vi "Logging Message Loop.vi"(8 "error in (no error)":errorcluster, 10 "Data Queue":refnum<queue>, 11 "Message Queues":T1) -> (0 "error out":errorcluster)   [LabVIEW 2023, in "Logging.lvlib"]
doc: "The message loop subVI to handle messages pertaining to logging data."
uses:
  Logging.lvlib
  support/Message Queue/All Message Queues.ctl
  support/Message Queue/Message Cluster.ctl
  Logging Configuration.ctl
  Logging State.ctl
  support/Message Queue/Enqueue Message (Single).vi
  <vilib>/Utility/error.llb/Error Cluster From Error Code.vi
  <vilib>/ErrorRing/Error Ring.xnode
  <vilib>/addons/_JKI.lib/REST Client/classes/REST Client/REST Client.lvclass
  support/Message Queue/Message Queue.lvlib
  <vilib>/addons/_JKI.lib/Serialization/JSON/JKI JSON Serialization.lvlib
panel:
  in  "CardId":string
  in  "City":string
  in  "Country":string="Poland"
  in  "FastAPI write route":string="/write_api"
  in  "FastAPI URI":string="http://localhost:80"
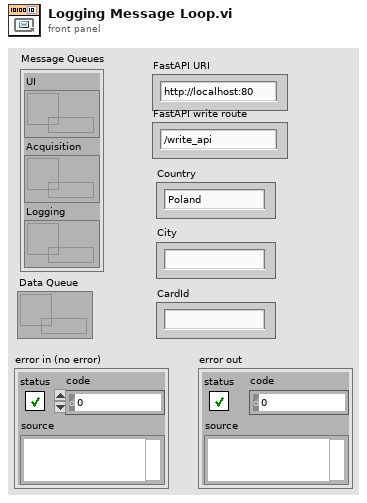
[diagram p1: front panel]
types:
  T1 = typedef "Message Queue.lvlib/All Message Queues.ctl" = cluster{"UI":refnum<queue>, "Acquisition":refnum<queue>, "Logging":refnum<queue>}
  T2 = typedef "Logging.lvlib/Logging Configuration.ctl" = cluster{"Log File Base Path":path, "TDMS File Reference":refnum<k34>}
  T3 = typedef "Logging.lvlib/Logging State.ctl" = enum16{"Idle", "Logging"}
  T4 = enum16{"open", "open or create", "create or replace", "create", "open (read-only)"}
  T5 = cluster{"Array":waveform(dbl)[], "Country":string, "City":string, "CardId":string}
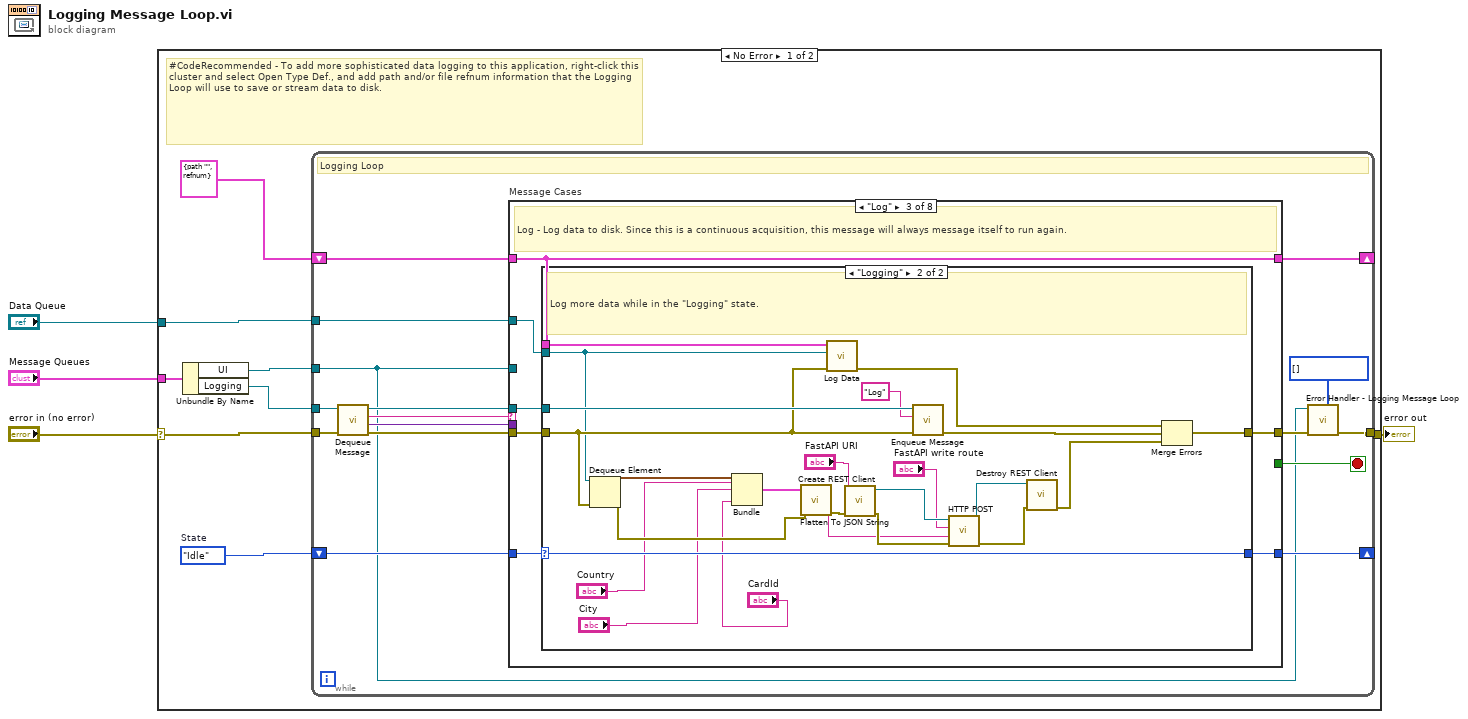
[diagram p0: block diagram]
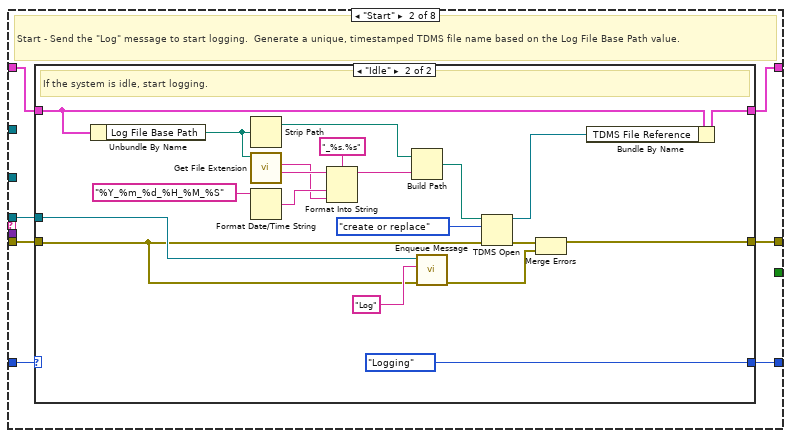
[diagram p3: hidden frame]
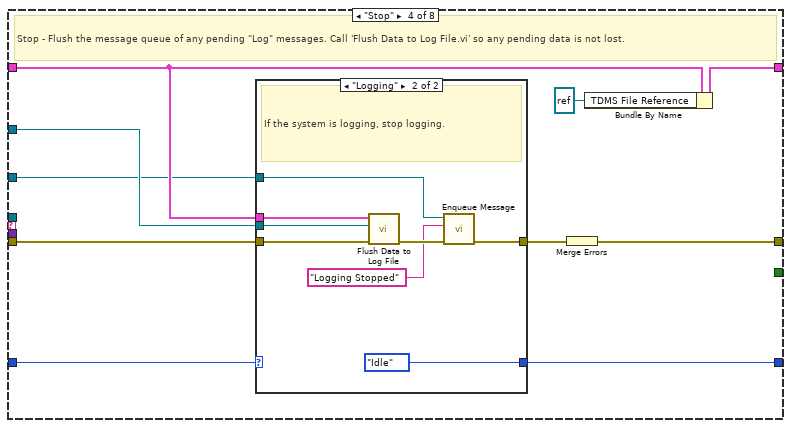
[diagram p6: hidden frame]
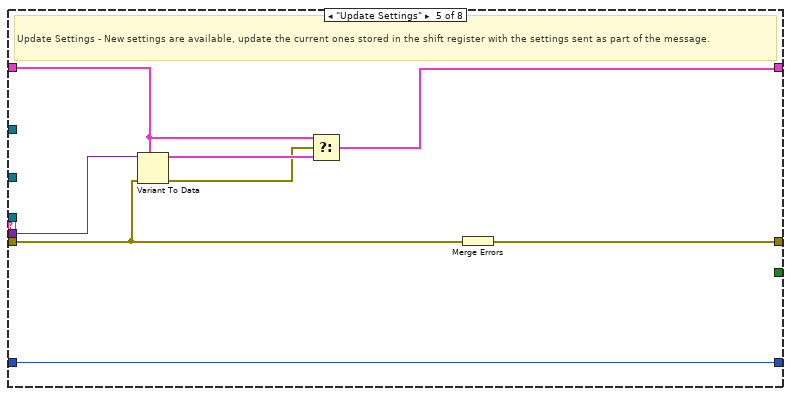
[diagram p8: hidden frame]
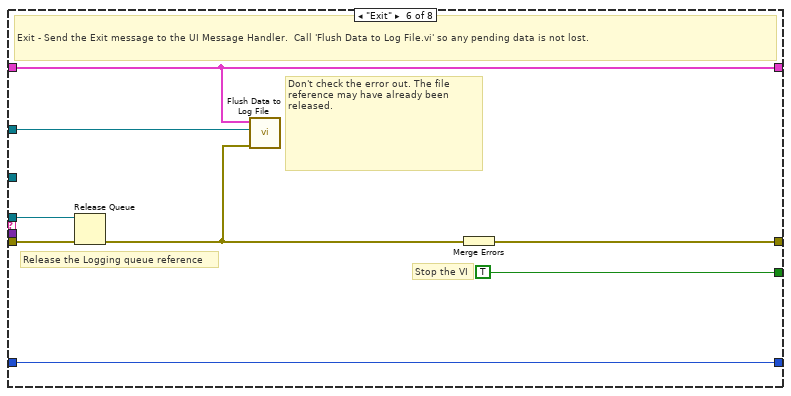
[diagram p9: hidden frame]
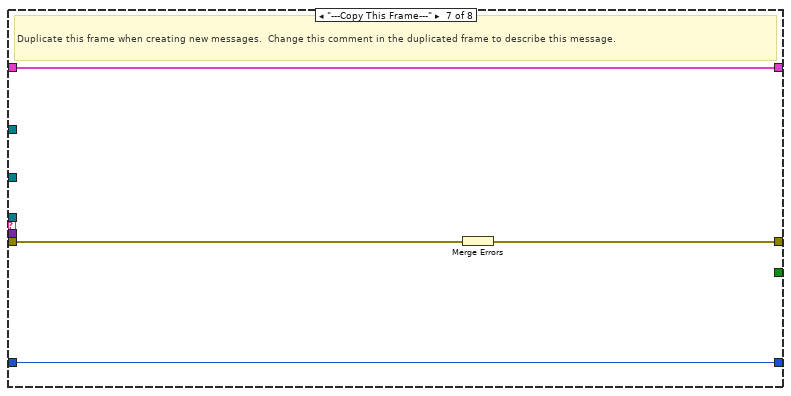
[diagram p10: hidden frame]
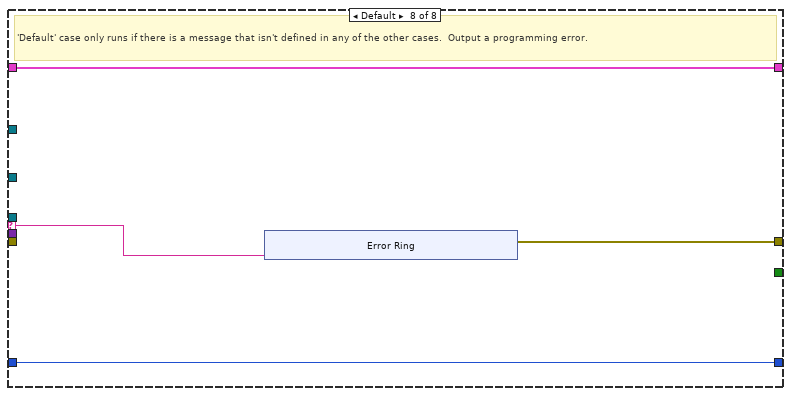
[diagram p11: hidden frame]
diagram:
  n1 = case shown="No Error" "error in (no error)" {
    selector: "error in (no error)" -> [w8 w146]
    tunnel: "Message Queues" -> [w12 _]
    tunnel: [w10 w146] -> w3
    tunnel: "Data Queue" -> [w7 _]
    frame No Error {
      w5 = Logging_State."Idle"  # State
      # "#CodeRecommended - To add more sophisticated data logging to this application, right-click this cluster and select Open Type Def., and add path and/or file refnum information that the Logging Loop will use to save or stream data to disk."
      n2 = Unbundle By Name(w12) -> ("UI"=w6:refnum<queue>, "Logging"=w11:refnum<queue>)
      n3 = while {
        tunnel: w11 -> [w20]
        shift-right: [w27] -> _
        shift-left: T2 {"Log File Base Path"=path "", "TDMS File Reference"=refnum} ("Logging Configuration") -> [w28]
        tunnel: w6 -> [w14]
        tunnel: w7 -> [w19]
        shift-right: [w17] -> _
        shift-left: w5 -> [w18]
        tunnel: w8 -> [w25]
        tunnel: [w16] -> w10
        stop <- w26 stop-if-true
        # "Logging Loop"
        n4 = call "Dequeue Message.vi"("error in (no error)"=w25, "Message Queue"=w20) -> ("error out"=w24:errorcluster, "Message Data"=w22:variant, "Message"=w23:string, "dup Message Queue"=w21:refnum<queue>)  [unwired: 6 in]
        n5 = case "Message Cases" shown="\"Log\"" w23 {
          selector: w23 -> [_ _ _ _ _ _ _ w135]
          tunnel: w21 -> [_ w37 w67 _ _ w127 _ _]
          tunnel: w24 -> [w30 w36 w65 w98 w116 w128 w134 _]
          tunnel: [w30 w38 w68 w104 w122 w129 w132 w136] -> w15
          tunnel: w28 -> [w31 w35 w64 w99 w120 w125 w133 w138]
          tunnel: [w31 w34 w64 w102 w117 w125 w133 w138] -> w27
          tunnel: [_ _ _ _ _ TRUE _ _] -> w26
          tunnel: w22 -> [_ _ _ _ w121 _ _ _]
          tunnel: w14 -> [_ _ _ w95 _ _ _ _]
          tunnel: w19 -> [_ _ w66 w100 _ w124 _ _]
          tunnel: w18 -> [w29 w33 w63 w97 w115 w123 w131 w137]
          tunnel: [w29 w32 w62 w96 w115 w123 w131 w137] -> w17
          frame "Initialize" {
            # "Initialize - gets called when first launched. Currently a no-op."
          }
          frame "Start" {
            # "Start - Send the \"Log\" message to start logging.  Generate a unique, timestamped TDMS file name based on the Log File Base Path value."
            n6 = case shown="\"Idle\"" w33 {
              selector: w33 -> [w40 _]
              tunnel: [w39 w43] -> w38
              tunnel: w37 -> [_ w44]
              tunnel: w36 -> [w39 w42]
              tunnel: w35 -> [w41 w45]
              tunnel: [w41 w47] -> w34
              tunnel: [w40 Logging_State."Logging" ("State")] -> w32
              frame "Logging" {
                # "The system is already logging. Ignore the \"Start\" message."
              }
              frame "Idle" {
                # "If the system is idle, start logging."
                n7 = Unbundle By Name(w45) -> ("Log File Base Path"=w60:path)
                n8 = Strip Path(path=w60) -> (stripped path=w57:path)  [unwired: 1 out]
                n9 = call <vilib>:"Get File Extension.vi"("file"=w60) -> ("filename without extension"=w58:string, "lowercase file extension"=w54:string)  [unwired: 6 in, 3 out]
                n10 = Format Date/Time String(time format string (%c)="%Y_%m_%d_%H_%M_%S") -> (date/time string=w55:string)  [unwired: 2 in]
                n11 = Format Into String(format string="_%s.%s", initial string=w58, w55, w54) -> (resulting string=w53:string)  [unwired: 1 in, 1 out]
                n12 = Build Path(base path=w57, name or relative path=w53) -> (appended path=w52:path)
                n13 = call-poly "Enqueue Message.vi"("error in (no error)"=w42, "Message"="Log", "Message Queue"=w44) -> ("error out"=w50:errorcluster)  [unwired: 7 in, 1 out]
                n14 = TDMS Open(8:w42, 10:T4."create or replace" ("operation (0:open)"), 11:w52) -> (0:w51:errorcluster, 3:w48:refnum<k34>)  [unwired: 4 in]
                n15 = Merge Errors(w51, w50) -> (w43:errorcluster)
                n16 = Bundle By Name(cluster=w45, "TDMS File Reference"=w48) -> (w47:T2)
              }
            }
          }
          frame "Log" {
            # "Log - Log data to disk. Since this is a continuous acquisition, this message will always message itself to run again."
            n17 = case shown="\"Logging\"" w63 {
              selector: w63 -> [w70 w88]
              tunnel: [w69 w94] -> w68
              tunnel: w67 -> [_ w92]
              tunnel: w66 -> [_ w83]
              tunnel: w65 -> [w69 w84]
              tunnel: w64 -> [_ w89]
              tunnel: [w70 w88] -> w62
              frame "Idle" {
                # "Ignore \"Log\" messages when the logging is idle."
              }
              frame "Logging" {
                # "Log more data while in the \"Logging\" state."
                n18 = Dequeue Element(queue=w83, error in (no error)=w84) -> (element=w75:waveform(dbl)[], error out=w76:errorcluster)  [unwired: 1 in, 2 out]
                n19 = Bundle("Array"=w75, "Country"="Country", "City"="City", "CardId"="CardId") -> (w74:T5)  [unwired: 1 in]
                n20 = call <vilib>:"Flatten To JSON String.vi"("error in (no error)"=w76, "Variant"=w74) -> ("error out"=w82:errorcluster, "JSON String"=w81:string)  [unwired: 8 in]
                n21 = call "Log Data.vi"("error in (no error)"=w84, "Data Queue"=w83, "Logging Configuration"=w89) -> ("error out"=w91:errorcluster)  [unwired: 8 in]
                n22 = call <vilib>:"Create REST Client.vi"("error in (no error)"=w82, "Base URL"="FastAPI URI") -> ("error out"=w85:errorcluster, "REST Client out"=w79:refnum<class "REST Client.lvclass">)  [unwired: 8 in]
                n23 = call-poly "Enqueue Message.vi"("error in (no error)"=w84, "Message"="Log", "Message Queue"=w92) -> ("error out"=w93:errorcluster)  [unwired: 7 in, 1 out]
                n24 = call-dynamic "HTTP POST.vi"("error in (no error)"=w85, "Request body"=w81, "Path"="FastAPI write route", "REST Client in"=w79) -> ("error out"=w86:errorcluster, "REST Client out"=w80:refnum<class "REST Client.lvclass">)  [unwired: 2 in, 4 out]
                n25 = call-dynamic "Destroy REST Client.vi"("error in (no error)"=w86, "REST Client in"=w80) -> ("error out"=w87:errorcluster)  [unwired: 9 in]
                n26 = Merge Errors(w91, w93, w87) -> (w94:errorcluster)
              }
            }
          }
          frame "Stop" {
            # "Stop - Flush the message queue of any pending \"Log\" messages. Call 'Flush Data to Log File.vi' so any pending data is not lost."
            n27 = case shown="\"Logging\"" w97 {
              selector: w97 -> [w105 _]
              tunnel: [w106 w109] -> w103
              tunnel: w100 -> [_ w113]
              tunnel: w99 -> [_ w112]
              tunnel: w98 -> [w106 w111]
              tunnel: [w105 Logging_State."Idle" ("State")] -> w96
              tunnel: w95 -> [_ w108]
              frame "Idle" {
                # "The system is already idle. Ignore the \"Stop\" message."
              }
              frame "Logging" {
                # "If the system is logging, stop logging."
                n28 = call "Flush Data to Log File.vi"("error in (no error)"=w111, "Data Queue"=w113, "Logging Configuration"=w112) -> ("error out"=w114:errorcluster)  [unwired: 8 in]
                n29 = call-poly "Enqueue Message.vi"("error in (no error)"=w114, "Message"="Logging Stopped", "Message Queue"=w108) -> ("error out"=w109:errorcluster)  [unwired: 7 in, 1 out]
              }
            }
            n30 = Merge Errors(w103) -> (w104:errorcluster)
            n31 = Bundle By Name(cluster=w99, "TDMS File Reference"=refnum<k34> refnum) -> (w102:T2)
          }
          frame "Update Settings" {
            # "Update Settings - New settings are available, update the current ones stored in the shift register with the settings sent as part of the message."
            n32 = Variant To Data(error in=w116, type=w120, Variant=w121) -> (data=w119:T2, error out=w118:errorcluster)
            n33 = Select(t=w120, s=w118, f=w119) -> (s? t:f=w117:T2)
            n34 = Merge Errors(w116) -> (w122:errorcluster)
          }
          frame "Exit" {
            # "Don't check the error out. The file reference may have already been released."
            # "Release the Logging queue reference"
            # "Stop the VI"
            # "Exit - Send the Exit message to the UI Message Handler.  Call 'Flush Data to Log File.vi' so any pending data is not lost."
            n35 = Release Queue(queue=w127, error in (no error)=w128) -> (error out=w126:errorcluster)  [unwired: 1 in, 2 out]
            n36 = call "Flush Data to Log File.vi"("error in (no error)"=w126, "Data Queue"=w124, "Logging Configuration"=w125) -> ()  [unwired: 8 in, 1 out]
            n37 = Merge Errors(w126) -> (w129:errorcluster)
          }
          frame "---Copy This Frame---" {
            # "Duplicate this frame when creating new messages.  Change this comment in the duplicated frame to describe this message."
            n38 = Merge Errors(w134) -> (w132:errorcluster)
          }
          frame Default {
            # "'Default' case only runs if there is a message that isn't defined in any of the other cases.  Output a programming error."
            n39 = xnode "Error Ring"("parameter 0"=w135) -> ("error out"=w136:errorcluster)
          }
        }
        n40 = call "Error Handler - Logging Message Loop.vi"("error in (no error)"=w15, "Ignore Errors (Runtime)"=i32[] [], "Message Queue"=w14) -> ("dup error in"=w16:errorcluster)  [unwired: 7 in, 1 out]
      }
    }
    frame Error {
    }
  }
  "error out" <- w3
